vi "TMC_Setup.vi"() -> ()   [LabVIEW 2019]
uses:
  TMC_Setup.ctl
panel:
  in  "TMC Torque Setup Cluster":T1={"flow control"=0, "stop bits"=10, "parity"=0, "data bits"=8, "baud rate"=9600, "VISA Torque Motor"="COM5"} {"data bits" min=5 max=8 step=1; "parity" items=["None", "Odd", "Even", "Mark", "Space"]; "stop bits" items=["1.0"=10, "1.5"=15, "2.0"=20]; "flow control" items=["None"=0, "XON/XOFF"=1, "RTS/CTS"=2, "DTR/DSR"=4]}
  # "Daten für Schnittstelle"
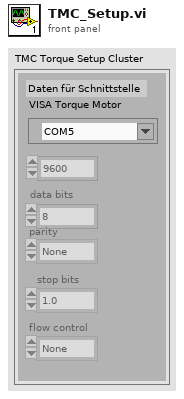
[diagram p1: front panel]
types:
  T1 = typedef "TMC_Setup.ctl" = cluster{"flow control":u16, "stop bits":u16, "parity":u16, "data bits":u16, "baud rate":u32, "VISA Torque Motor":refnum<visa-resource-name>}
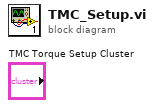
[diagram p0: block diagram]
diagram:
